vi "Read_data_from_Agilent.vi"(8 "stop bits (10: 1 bit)":u16(ring)=10 items=["1.0"=10, "1.5"=15, "2.0"=20], 9 "parity (0:none)":enum16{"None", "Odd", "Even", "Mark", "Space"}(ring), 10 "data bits (8)":u16=8 min=5 max=8 step=1, 11 "baud rate (9600)":u32=9600) -> (0 "read buffer":string)   [LabVIEW 2022 SP3]
uses:
  <vilib>/Instr/_visa.llb/VISA Configure Serial Port (Instr).vi
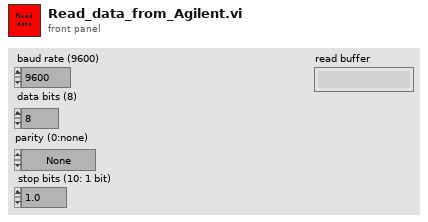
[diagram p1: front panel]
types:
  T1 = enum16{"open", "replace", "create", "open or create", "replace or create", "replace or create with confirmation"}
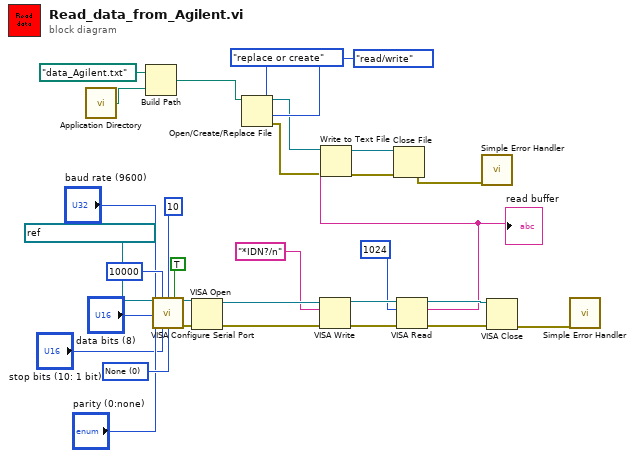
[diagram p0: block diagram]
diagram:
  w19 = u16 0 items=["None", "XON/XOFF", "RTS/CTS", "XON/XOFF & RTS/CTS", "DTR/DSR", "XON/XOFF & DTR/DSR"] ("flow control (0:none)")
  n1 = call <vilib>:"Application Directory.vi"() -> ("Application Directory"=w11:path)
  n2 = Build Path(base path=path "data_Agilent.txt", name or relative path=w11) -> (appended path=w13:path)
  n3 = call-poly "VISA Configure Serial Port"("VISA resource name"=refnum<visa-resource-name> "GPIB0::10::INSTR", "timeout (10sec)"=u32 10000, "termination char\n(0xA = '\\n' = LF)"=u8 10 ("termination char\n(0xA = '\\n' = LF)"), "Enable Termination\nChar (T)"=TRUE ("Enable Termination\nChar (T)"), "baud rate (9600)"="baud rate (9600)", "data bits (8)"="data bits (8)", "parity (0:none)"="parity (0:none)", "stop bits (10: 1 bit)"="stop bits (10: 1 bit)", "flow control (0:none)"=w19) -> ("VISA resource name out"=w21:refnum<visa-resource-name>, "error out"=w20:errorcluster)  [unwired: 5 in]
  n4 = VISA Open(error in (no error)=w20, VISA resource name=w21) -> (VISA resource name=w31:refnum<visa-resource-name>, error out=w26:errorcluster)  [unwired: 3 in]
  n5 = Open/Create/Replace File(file path (use dialog)=w13, operation (0:open)=T1."replace or create", access (0:read/write)=enum16{"read/write", "read-only", "write-only"}."read/write") -> (refnum out=w10:refnum<file>, error out=w6:errorcluster)  [unwired: 3 in, 1 out]
  n6 = VISA Write(VISA resource name=w31, write buffer="*IDN?/n", error in (no error)=w26) -> (VISA resource name out=w30:refnum<visa-resource-name>, error out=w27:errorcluster)  [unwired: 1 out]
  n7 = VISA Read(VISA resource name=w30, byte count=u32 1024, error in (no error)=w27) -> (VISA resource name out=w29:refnum<visa-resource-name>, read buffer=w9:string, error out=w28:errorcluster)  [unwired: 1 out]
  "read buffer" <- w9
  n8 = Write to Text File(file (use dialog)=w10, text=w9, error in=w6) -> (refnum out=w8:refnum<file>, error out=w7:errorcluster)  [unwired: 1 in, 1 out]
  n9 = Close File(refnum=w8, error in=w7) -> (error out=w5:errorcluster)  [unwired: 1 out]
  n10 = call <vilib>:"Simple Error Handler.vi"("error in (no error)"=w5) -> ()  [unwired: 4 in, 5 out]
  n11 = VISA Close(VISA resource name=w29, error in (no error)=w28) -> (error out=w23:errorcluster)
  n12 = call <vilib>:"Simple Error Handler.vi"("error in (no error)"=w23) -> ()  [unwired: 4 in, 5 out]
